vi "Lab1.vi"() -> ()   [LabVIEW 2014]
uses:
  <vilib>/Instr/_visa.llb/VISA Configure Serial Port (Instr).vi
panel:
  in  "file (use dialog)":path
  in  "Timeout [ms]":u32=5000
  in  "Stop everything":bool
  in  "Send request":bool
  out "Answer":string
  in  "Request":string
  in  "parity (0:none)":enum16{"None", "Odd", "Even", "Mark", "Space"}(ring)
  in  "data bits (8)":u16=8 min=5 max=8 step=1
  in  "baud rate (9600)":u32=9600
  in  "VISA resource name":refnum<visa-resource-name>
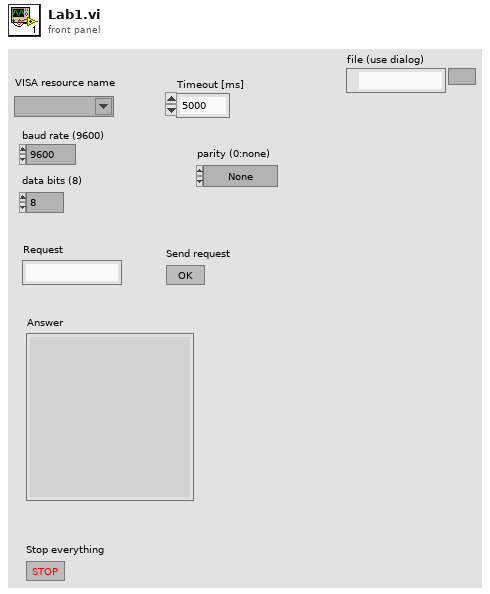
[diagram p1: front panel]
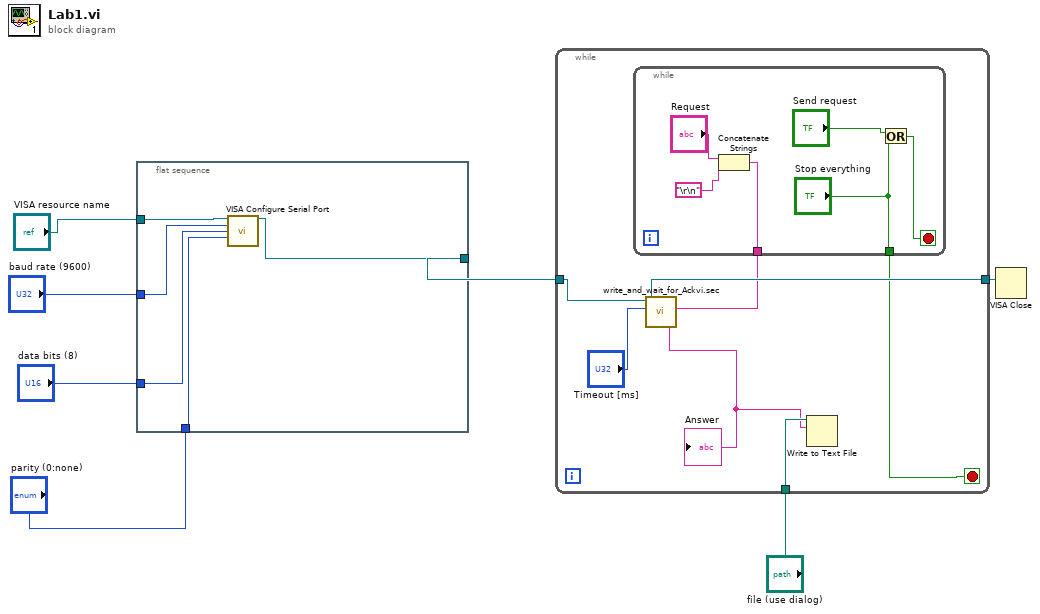
[diagram p0: block diagram]
diagram:
  n1 = flat-sequence {
    tunnel: "VISA resource name" -> [w12]
    tunnel: "parity (0:none)" -> [w11]
    tunnel: "data bits (8)" -> [w10]
    tunnel: "baud rate (9600)" -> [w9]
    tunnel: [w8] -> w3
    frame #0 {
      n2 = call-poly "VISA Configure Serial Port"("VISA resource name"=w12, "baud rate (9600)"=w9, "data bits (8)"=w10, "parity (0:none)"=w11) -> ("VISA resource name out"=w8:refnum<visa-resource-name>)  [unwired: 10 in, 1 out]
    }
  }
  n3 = while {
    tunnel: w3 -> [w19]
    tunnel: [w18] -> w2
    tunnel: "file (use dialog)" -> [w14]
    stop <- w16 stop-if-true
    n4 = while {
      tunnel: [w23] -> w17
      tunnel: ["Stop everything"] -> w16
      stop <- w20 stop-if-true
      n5 = Concatenate Strings("Request", "\r\n") -> (w23:string)
      n6 = Or(x="Send request", y="Stop everything") -> (x .or. y?=w20:bool)
    }
    n7 = call "write_and_wait_for_Ackvi.sec"("request"=w17, "Timeout [ms]"="Timeout [ms]", "VISA resource name"=w19) -> ("result"=w13:string, "VISA resource name out"=w18:refnum<visa-resource-name>)  [unwired: 4 in, 1 out]
    "Answer" <- w13
    n8 = Write to Text File(file (use dialog)=w14, text=w13) -> ()  [unwired: 2 in, 3 out]
  }
  n9 = VISA Close(VISA resource name=w2) -> ()  [unwired: 1 in, 1 out]
